vi "Single Mouse Test.vi"() -> ()   [LabVIEW 2011]
uses:
  <vilib>/vision/NI_Vision_Development_Module.lvlib
panel:
  in  "Size & Tolerance":T1={"X Size"=3, "Y Size"=3, "% Tolerance"=40}
  out "Center Line":dbl[](graph)
  out "Right Left":T2(graph)
  out "Right Histogram":T3(graph)
  out "Left Histogram":T3(graph)
  out "dAngle/dt":dbl(graph)
  out "Angle":dbl(graph)
  out "Just Mouse":T4(plugin-control)
  out "Image #":i32
  out "Image":T4(plugin-control)
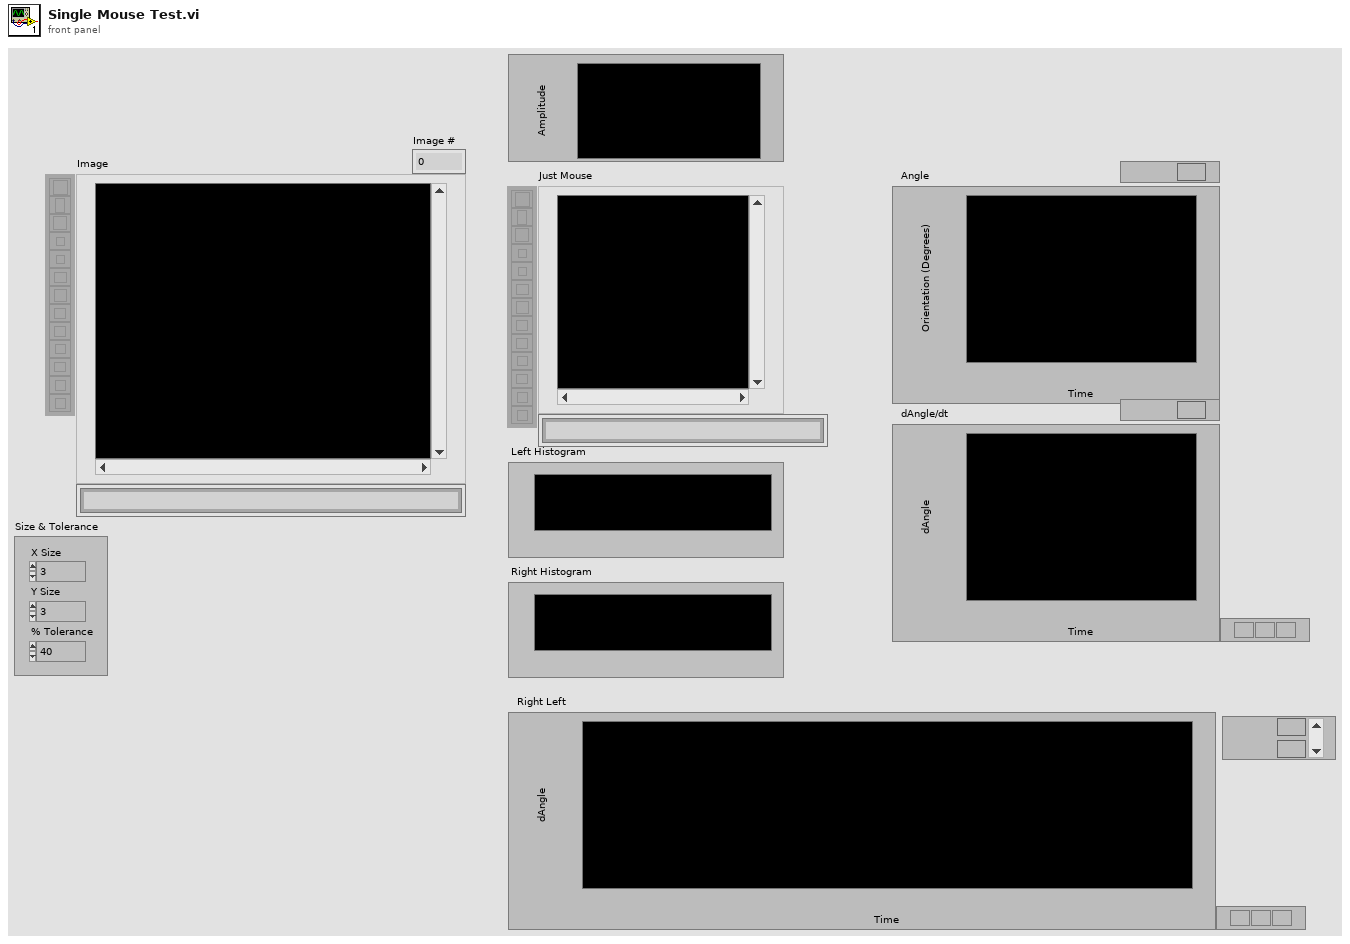
[diagram p1: front panel]
types:
  T1 = cluster{"X Size":i32, "Y Size":i32, "% Tolerance":i32}
  T2 = cluster{"Mean Left Value":sgl, "Mean Right Value":sgl}
  T3 = cluster{"Starting Value":sgl, "Incremental Value":sgl, "Histogram":u32[]}
  T4 = typedef "IMAQ Image.ctl" = refnum<image>
  T5 = typedef "Image Type" = u32
  T6 = cluster{"Area":dbl, "Number of Holes":dbl, "Bounding Rect":cluster{"Left":dbl, "Top":dbl, "Right":dbl, "Bottom":dbl}, "Center of Mass":cluster{"X":dbl, "Y":dbl}, "Orientation":dbl, "Dimensions":cluster{"Width":dbl, "Height":dbl}}[]
  T7 = cluster{"Area":dbl, "Number of Holes":dbl, "Bounding Rect":cluster{"Left":dbl, "Top":dbl, "Right":dbl, "Bottom":dbl}, "Center of Mass":cluster{"X":dbl, "Y":dbl}, "Orientation":dbl, "Dimensions":cluster{"Width":dbl, "Height":dbl}}
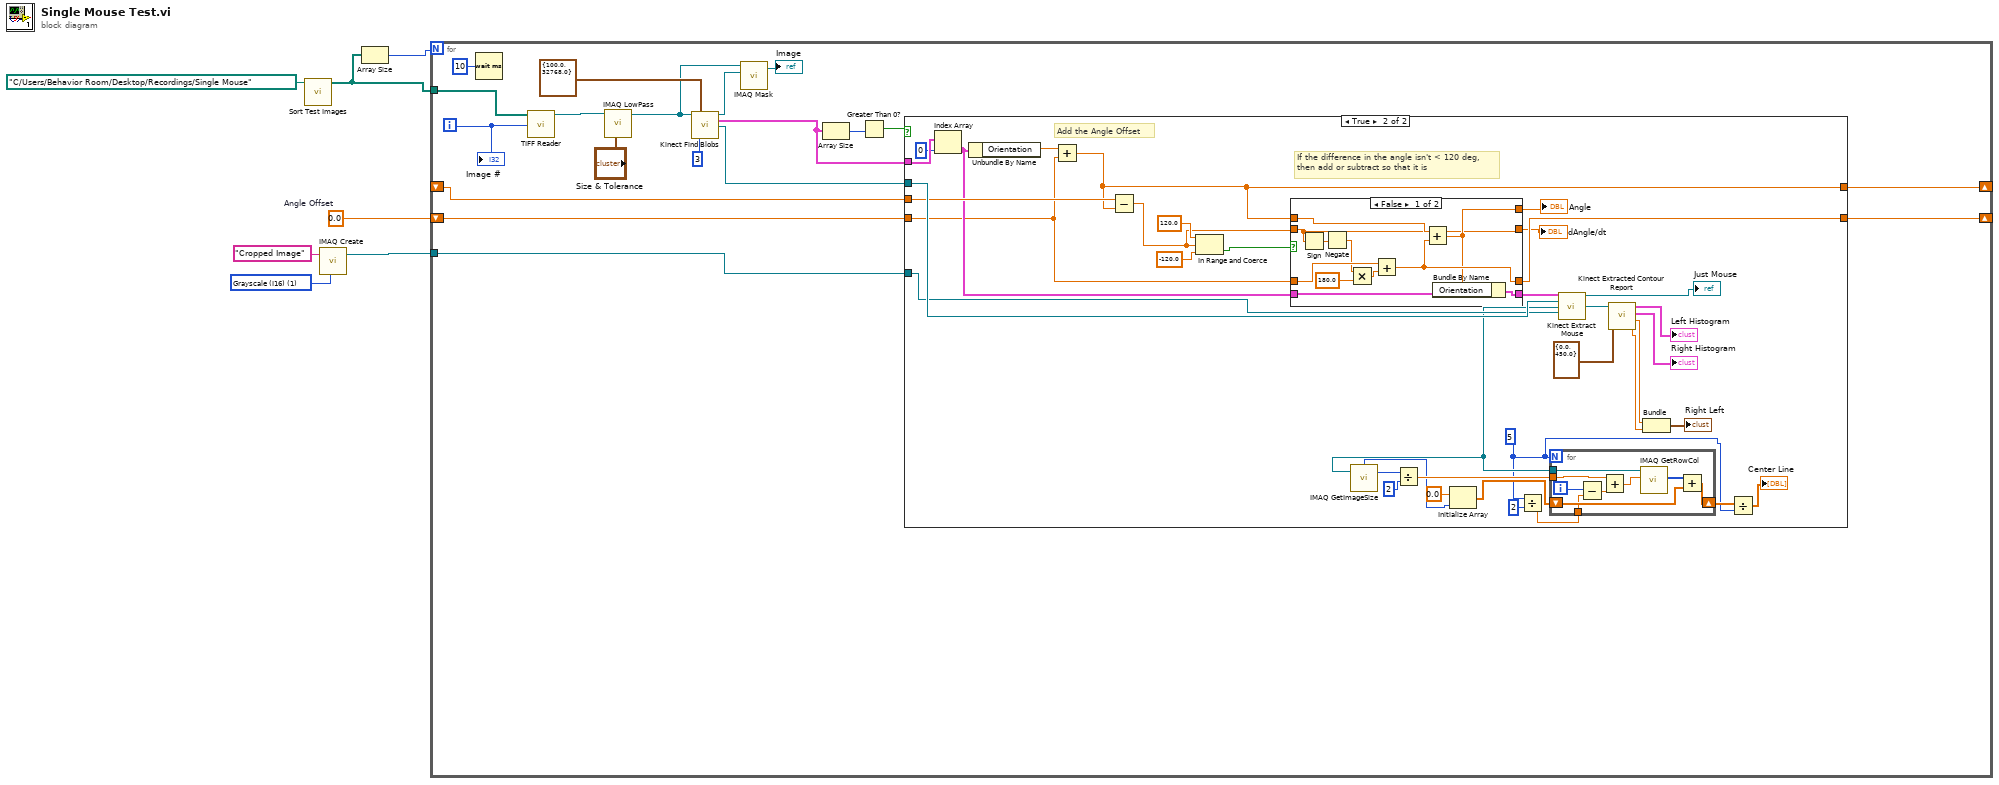
[diagram p0: block diagram]
diagram:
  w2 = 0.0  # Angle Offset
  w4 = T5 1 items=["Grayscale (U8)", "Grayscale (I16)", "Grayscale (SGL)", "Complex (CSG)", "RGB (U32)", "HSL (U32)", "RGB (U64)", "Grayscale (U16)"] ("Image Type")
  n1 = call "Sort Test Images.vi"("path"=path "C:/Users/Behavior Room/Desktop/Recordings/Single Mouse") -> ("Array"=w6:path[])  [unwired: 10 in]
  n2 = call "IMAQ Create"("Image Name"="Cropped Image", "Image Type"=w4) -> ("New Image"=w3:T4)  [unwired: 3 in, 1 out]
  n3 = Array Size(array=w6) -> (size(s)=w7:i32)
  n4 = for {
    N: w7 -> [_]
    tunnel: w6 -> [w26]
    tunnel: w3 -> [w18]
    shift-right: [w15] -> _
    shift-left: _ -> [w14]
    shift-right: [w12] -> _
    shift-left: w2 -> [w13]
    i -> [w25]
    n5 = Wait (ms)(milliseconds to wait=u32 10) -> ()  [unwired: 1 out]
    n6 = call "TIFF Reader.vi"("index"=w25, "Array"=w26) -> ("Image Out"=w10:T4)  [unwired: 9 in]
    n7 = call "IMAQ LowPass"("Image Src"=w10, "Size & Tolerance"="Size & Tolerance") -> ("Image Dst Out"=w9:T4)  [unwired: 5 in, 1 out]
    n8 = call "Kinect Find Blobs.vi"("Image Src"=w9, "Range"=cluster{"Lower value":sgl, "Upper value":sgl} {"Lower value"=100.0, "Upper value"=32768.0}, "Number of Erosion"=3) -> ("Masked Image Out"=w16:T4, "Particle Reports (Pixels)"=w19:T6, "Src Image Out"=w17:T4)  [unwired: 10 in]
    n9 = call "IMAQ Mask"("Image Mask"=w16, "Image Src"=w9) -> ("Image Dst Out"=→"Image":T4)  [unwired: 3 in, 1 out]
    n10 = Array Size(array=w19) -> (size(s)=w21:i32)
    n11 = Greater Than 0?(x=w21) -> (x > 0?=w20:bool)
    n12 = case shown="True" w20 {
      tunnel: w19 -> [_ w63]
      tunnel: w17 -> [_ w61]
      tunnel: w18 -> [_ w60]
      tunnel: [w28 w49] -> w15
      tunnel: w14 -> [w28 w59]
      tunnel: w13 -> [w27 w51]
      tunnel: [w27 w50] -> w12
      frame False {
      }
      frame True {
        w29 = 5
        # "If the difference in the angle isn't < 120 deg,\nthen add or subtract so that it is"
        # "Add the Angle Offset"
        n13 = Index Array(array=w63, index=0) -> (element=w54:T7)
        n14 = Unbundle By Name(w54) -> ("Orientation"=w55:dbl)
        n15 = Add(x=w55, y=w51) -> (x+y=w49:dbl)
        n16 = Subtract(x=w59, y=w49) -> (x-y=w52:dbl)
        n17 = In Range and Coerce(upper limit=120.0, x=w52, lower limit=-120.0 ("upper limit")) -> (In Range?=w56:bool)  [unwired: 1 out]
        n18 = case shown="False" w56 {
          tunnel: w54 -> [w80 w87]
          tunnel: [w79 w87] -> w53
          tunnel: w52 -> [w73 w84]
          tunnel: [w81 w86] -> w50
          tunnel: w51 -> [w83 w86]
          tunnel: w49 -> [w82 w85]
          tunnel: [w74 w85] -> w48
          tunnel: [w73 w84] -> w47
          frame False {
            n19 = Sign(1:w73) -> (0:w78:dbl)
            n20 = Negate(x=w78) -> (-x=w77:dbl)
            n21 = Multiply(x=w77, y=180.0) -> (x*y=w76:dbl)
            n22 = Add(x=w83, y=w76) -> (x+y=w81:dbl)
            n23 = Add(x=w82, y=w81) -> (x+y=w74:dbl)
            n24 = Bundle By Name(cluster=w80, "Orientation"=w74) -> (w79:T7)
          }
          frame True {
          }
        }
        "Angle" <- w48
        "dAngle/dt" <- w47
        n25 = Divide(x=w29, y=2) -> (x/y=w35:dbl)
        n26 = call "Kinect Extract Mouse.vi"("Particle Report"=w53, "Image Src"=w61, "Image Dst"=w60) -> ("Cropped Image Out"=w40:T4)  [unwired: 11 in, 1 out]
        "Just Mouse" <- w40
        n27 = call "IMAQ GetImageSize"("Image"=w40) -> ("Y Resolution"=w39:i32, "X Resolution"=w33:i32)  [unwired: 3 in, 1 out]
        n28 = Divide(x=w39, y=2) -> (x/y=w37:dbl)
        n29 = Initialize Array(0.0 ("element"), w33) -> (w32:dbl[])
        n30 = for {
          N: w29 -> [_]
          tunnel: w40 -> [w72]
          tunnel: w37 -> [w68]
          shift-right: [w70] -> w31
          shift-left: w32 -> [w69]
          tunnel: w35 -> [w64]
          i -> [w66]
          n31 = Subtract(x=w66, y=w64) -> (x-y=w65:dbl)
          n32 = Add(x=w68, y=w65) -> (x+y=w67:dbl)
          n33 = call "IMAQ GetRowCol"("Image"=w72, "Number"=w67) -> ("Pixels (I16)"=w71:i16[])  [unwired: 4 in, 4 out]
          n34 = Add(x=w71, y=w69) -> (x+y=w70:dbl[])
        }
        n35 = call "Kinect Extracted Contour Report.vi"("Interval Range"=cluster{"Minimum":sgl, "Maximum":sgl} {"Minimum"=0.0, "Maximum"=450.0}, "Image"=w40) -> ("Mean Right Value"=w41:sgl, "Mean Left Value"=w42:sgl, "Right Histogram"=→"Right Histogram":T3, "Left Histogram"=→"Left Histogram":T3)  [unwired: 6 in]
        n36 = Bundle("Mean Left Value"=w42, "Mean Right Value"=w41) -> (→"Right Left":T2)  [unwired: 1 in]
        n37 = Divide(x=w31, y=w29) -> (x/y=→"Center Line":dbl[])
      }
    }
    "Image #" <- w25
  }
